vi "含算法图_new3.vi"() -> ()   [LabVIEW 2014]
uses:
  <vilib>/Instr/_visa.llb/VISA Configure Serial Port (Instr).vi
  test_last/Debug/test_last.dll
panel:
  out "数值 5":u8
  out "数值":dbl
  in  "?":enum32{"串口助手", "姿态界面", "曲线显示", "图像显示", "使用说明"}(tab)=enum."图像显示"
  in  "单选按钮":T1(radio)
  in  "?":bool
  out "接受数据个数":u32
  out "发送数据个数":u32
  in  "?":bool
  out "?":bool
  in  "?":bool
  in  "停止位":u16(ring)=10 items=["1.0"=10, "1.5"=15, "2.0"=20]
  in  "com口":refnum<visa-resource-name>="COM2"
  in  "波特率":u32(ring)=115200 items=["4800"=4800, "9600"=9600, "14400"=14400, "19200"=19200, "38400"=38400, "56000"=56000, "57600"=57600, "115200"=115200]
  in  "数据位数":u16(ring)=8 caption="数据位" items=["5"=5, "6"=6, "7"=7, "8"=8]
  in  "校验位":u16(ring) items=["None", "Odd", "Even", "Mark", "Space"]
  in  "?":string
  out "?":string
  in  "?":bool=TRUE
  out "数值 3":dbl
  out "数值 2":u8
  in  "舵机":sgl(slide) scale=5.0..10.0
  in  "电机":sgl(slide) scale=0.0..100.0
  out "数值 4":dbl
  out "波形图表":cluster{sgl, sgl}[](graph)
  in  "白界":u8=120
  in  "黑界":u8=100
  in  "列数":i32=190
  in  "行数":i32=130
  out "?":string
  out "new picture":picture caption="新图片"
  out "一帧数据数":i32
  in  "?":bool=TRUE
  # "数据类型"
  # "串口配置"
  # "串口号"
  # "上位机通信协议及功能介绍"
  # "功能1：串口助手"
  # "HEX:字符串显示\nDefault:十进制显示\nuint8:十六进制显示\nint32:输入字符串“in32”+BYTE1+BYTE2+BYTE3+BYTE4\nfloat:输入字符串“flot”+BYTE1+BYTE2+BYTE3+BYTE4\nuint32:输入字符串“ui32”+BYTE1+BYTE2+BYTE3+BYTE4"
  # "功能2：姿态界面"
  # "舵机发送：0x08+0x00+0x02+0x03+BYTE1+BYTE2+BYTE3+BYTE4\n电机发送：0X08+0X01+0X02+0X03+BYTE1+BYTE2+BYTE3+BYTE4"
  # "功能3：曲线显示"
  # "曲线1：“lin1”+BYTE1+BYTE2+BYTE3+BYTE4(发送一个float数据)\n曲线2：“lin2”+BYTE1+BYTE2+BYTE3+BYTE4(发送一个float数据)"
  # "功能4：图像显示"
  # "图像：发送字符串“image”+图像数组"
  # "LJ     HNU"
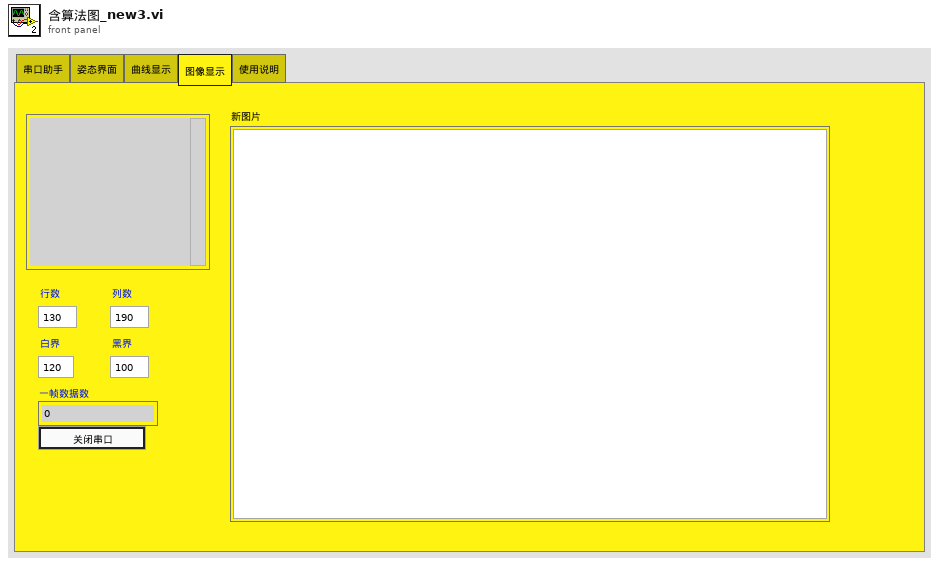
[diagram p1: front panel]
types:
  T1 = enum32{"uint8", "uint32", "HEX", "int8", "int32", "float", "Default"}
  T2 = typedef "imagedata.ctl" = cluster{"image type":i32, "image depth":i32, "image":u8[], "mask":u8[], "colors":u32[], "Rectangle":cluster{"left":i16, "top":i16, "right":i16, "bottom":i16}}
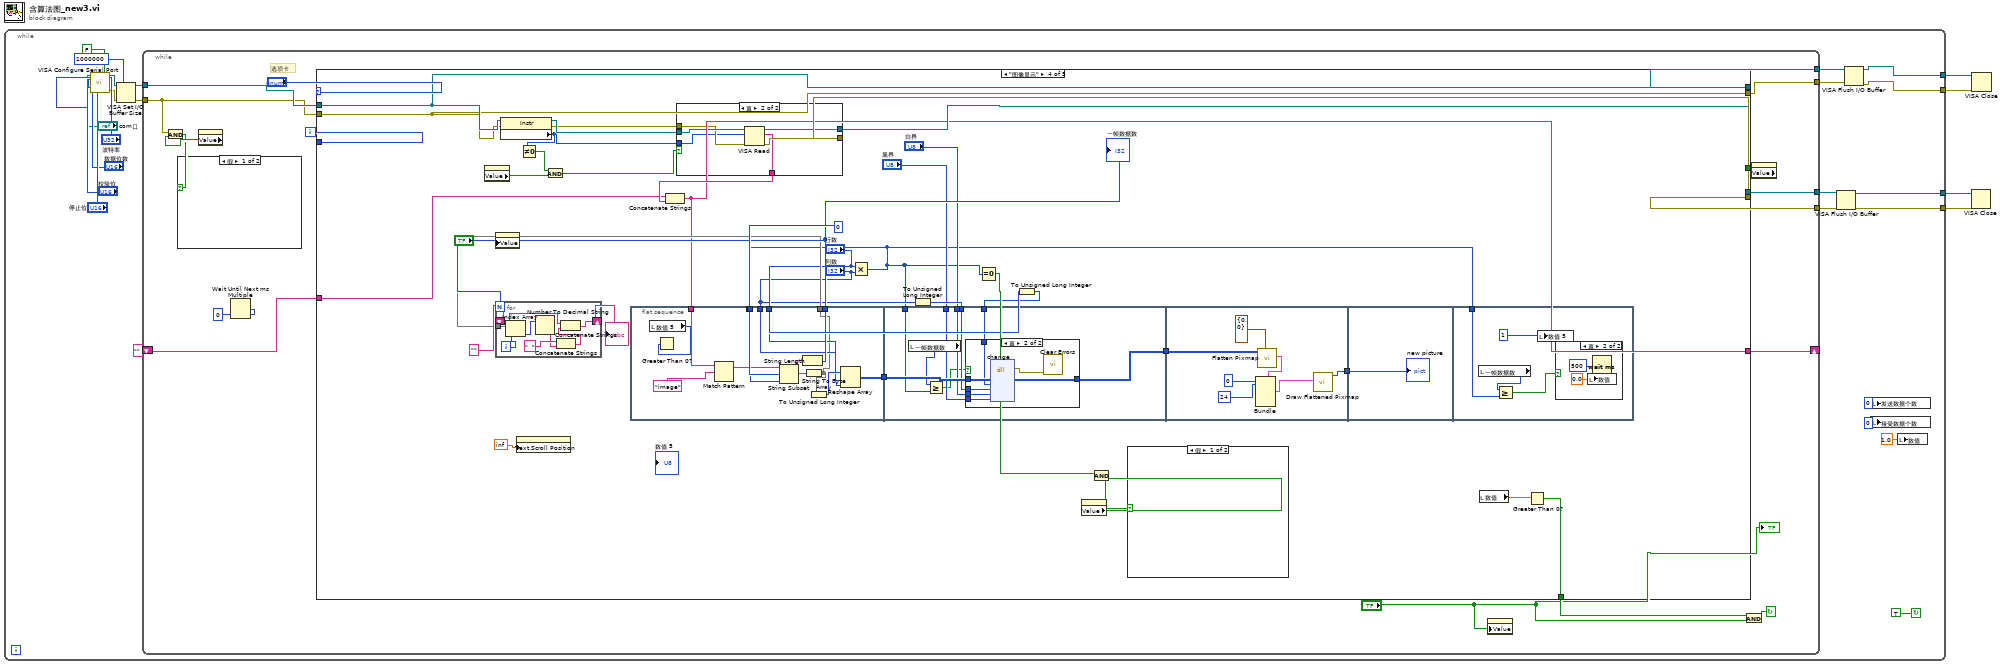
[diagram p0: block diagram]
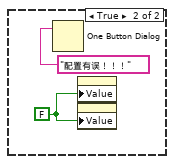
[diagram p2: hidden frame]
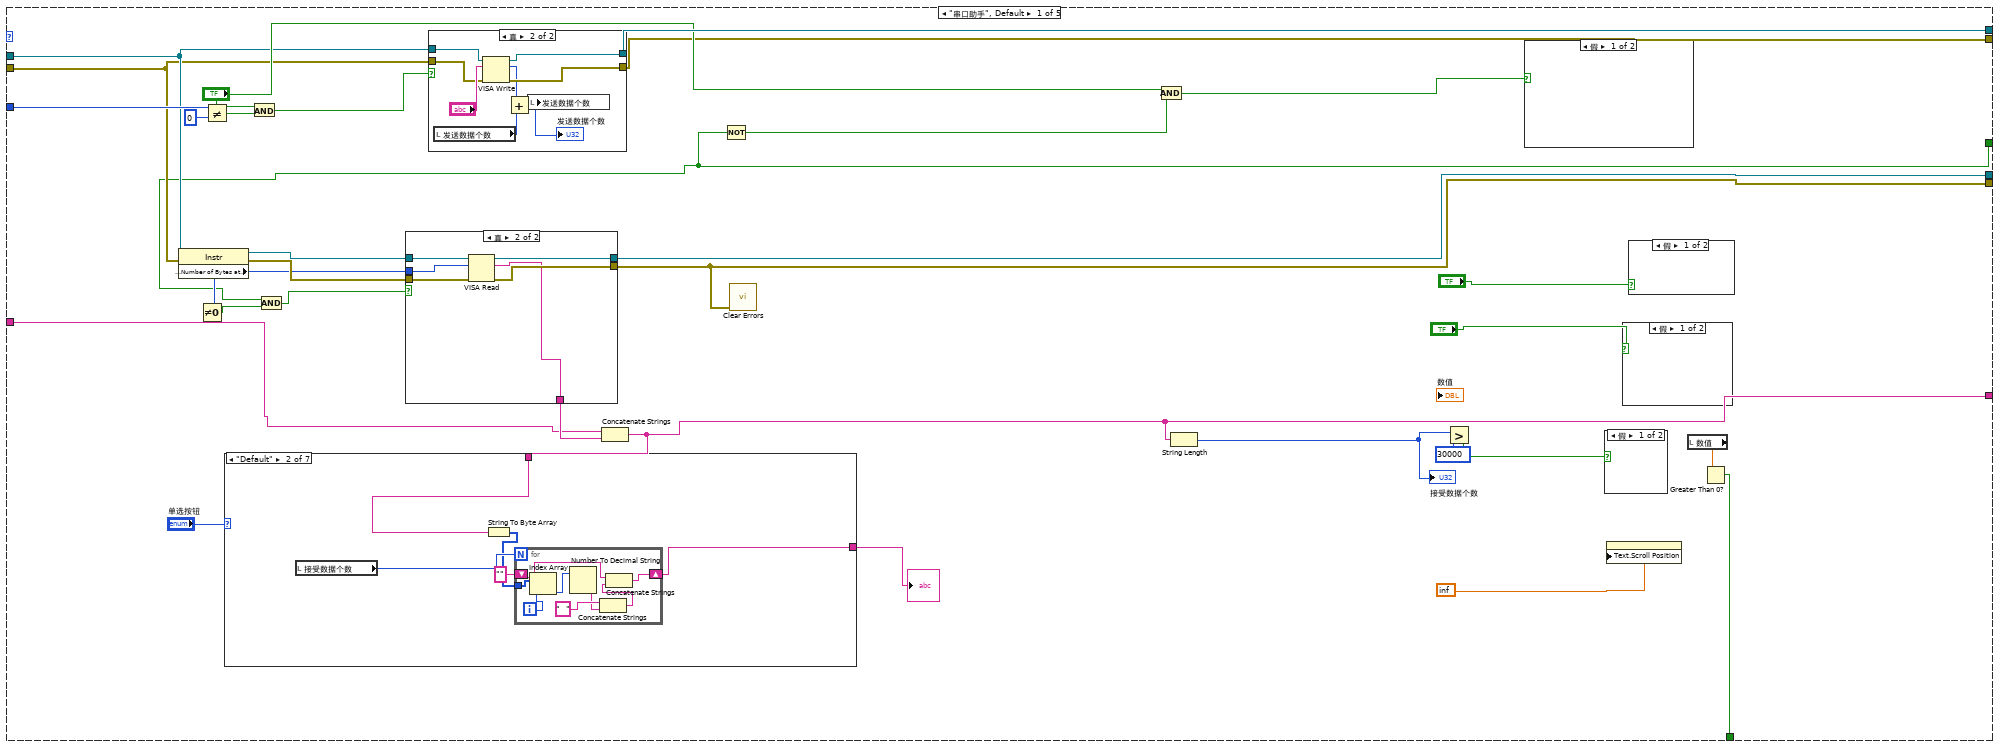
[diagram p3: hidden frame]
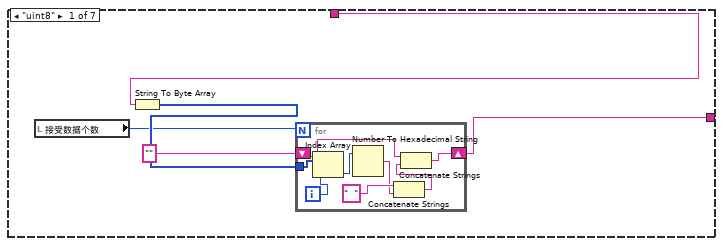
[diagram p4: hidden frame]
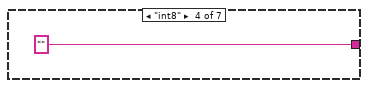
[diagram p6: hidden frame]
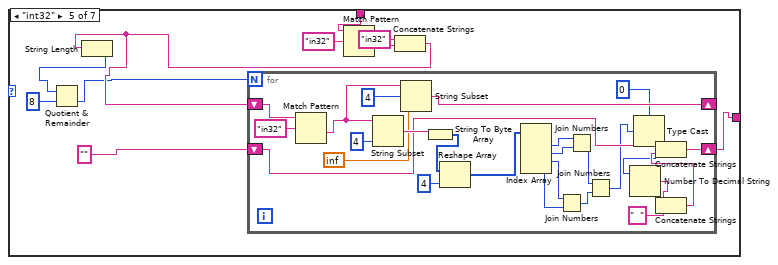
[diagram p7: hidden frame]
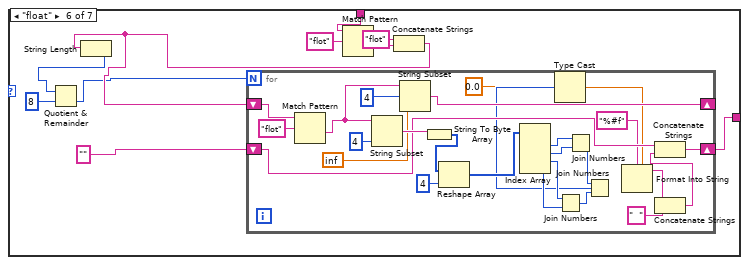
[diagram p8: hidden frame]
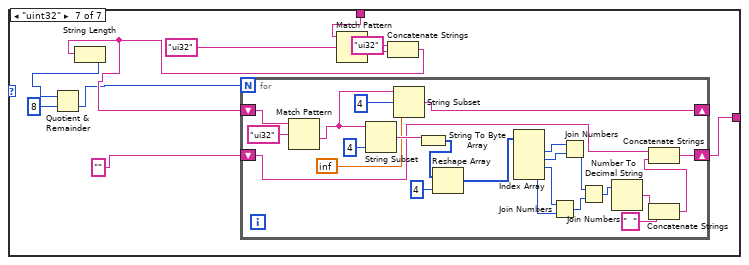
[diagram p9: hidden frame]
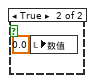
[diagram p10: hidden frame]
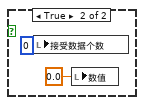
[diagram p11: hidden frame]
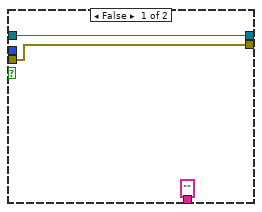
[diagram p12: hidden frame]
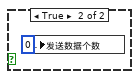
[diagram p13: hidden frame]
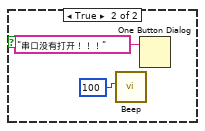
[diagram p14: hidden frame]
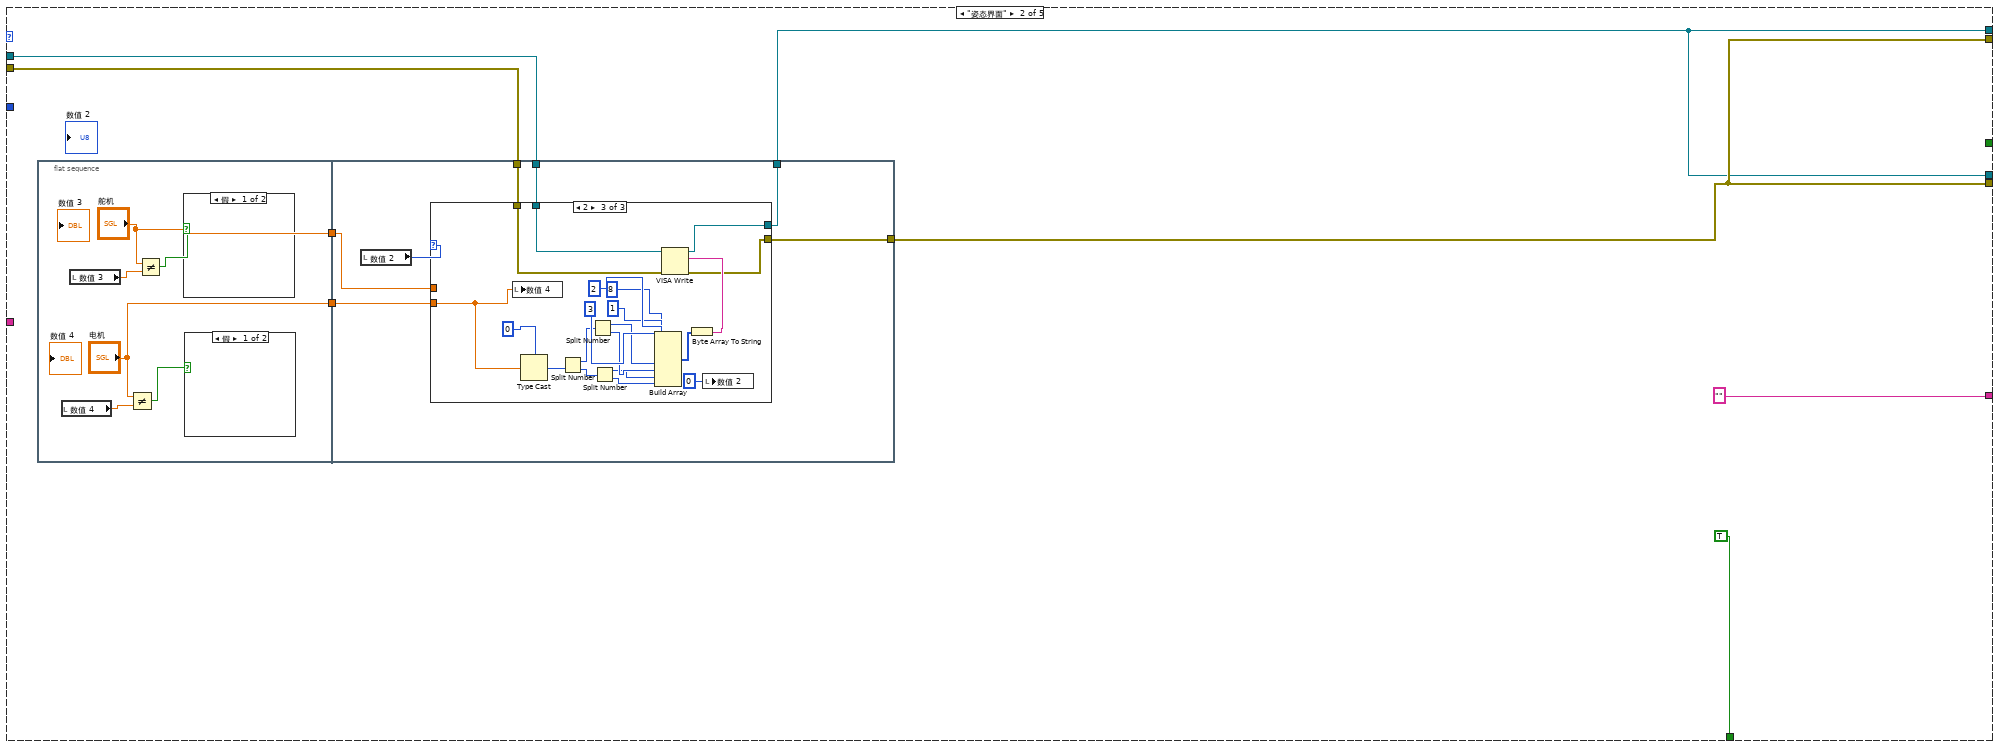
[diagram p16: hidden frame]
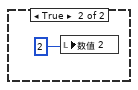
[diagram p17: hidden frame]
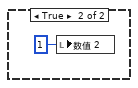
[diagram p18: hidden frame]
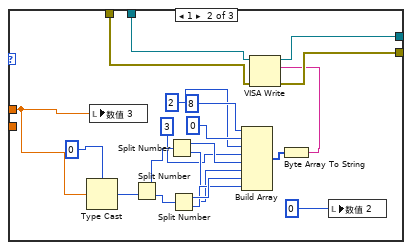
[diagram p20: hidden frame]
diagram:
  n1 = while {
    tunnel: [w9] -> w4
    tunnel: [w8] -> w3
    tunnel: [w7] -> w2
    tunnel: [w6] -> w1
    stop <- TRUE continue-if-true
    n2 = call-poly "VISA Configure Serial Port"("VISA resource name"="com口", "Enable Termination\nChar (T)"=FALSE ("Enable Termination\nChar (T)"), "baud rate (9600)"="波特率", "data bits (8)"="数据位数", "parity (0:none)"="校验位", "stop bits (10: 1 bit)"="停止位") -> ("VISA resource name out"=w22:refnum<visa-resource-name>, "error out"=w20:errorcluster)  [unwired: 8 in]
    n3 = VISA Set I/O Buffer Size(VISA resource name=w22, size (4096)=1000000, error in (no error)=w20) -> (VISA resource name out=w15:refnum<visa-resource-name>, error out=w5:errorcluster)  [unwired: 1 in]
    n4 = while {
      tunnel: w15 -> [w43]
      tunnel: w5 -> [w32]
      shift-right: [w42] -> _
      shift-left: "" -> [w41]
      tunnel: [w36] -> w14
      tunnel: [w33] -> w13
      tunnel: [w35] -> w12
      tunnel: [w34] -> w11
      i -> [w45]
      stop <- w39 continue-if-true
      # "选项卡"
      n5 = property class="Bool (严格)"() -> ("Value"=w31:bool)  [unwired: 2 in, 2 out]
      n6 = And(x=w32, y=w31) -> (x .and. y?=w30:bool)
      n7 = case shown="假" w30 {
        frame False {
        }
        frame True {
          w46 = FALSE
          n8 = One Button Dialog(message="配置有误！！！" ("消息")) -> ()  [unwired: 1 in, 1 out]
          n9 = property class="Bool (严格)"("Value"=w46) -> ()  [unwired: 2 in, 2 out]
          n10 = property class="Bool (严格)"("Value"=w46) -> ()  [unwired: 2 in, 2 out]
        }
      }
      n11 = Wait Until Next ms Multiple(millisecond multiple=u32 0 ("毫秒倍数")) -> ()  [unwired: 1 out]
      n12 = property class="Bool (严格)"("Value"="?") -> ()  [unwired: 2 in, 2 out]
      n13 = property class="Bool (严格)"() -> ("Value"=w37:bool)  [unwired: 2 in, 2 out]
      n14 = case shown="\"图像显示\"" "?" {
        tunnel: [w79 w237 w324 w416 w484] -> w36
        tunnel: [w49 w238 w323 w395 w483] -> w33
        tunnel: w45 -> [w78 _ _ _ _]
        tunnel: w43 -> [w70 w241 w331 w416 w484]
        tunnel: w32 -> [w69 w240 w330 w395 w483]
        tunnel: w37 -> [w59 _ _ _ _]
        tunnel: [w65 w237 w324 w415 w484] -> w35
        tunnel: [w48 w238 w323 w417 w483] -> w34
        tunnel: [w50 "" "" w384 ""] -> w42
        tunnel: w41 -> [w60 _ w319 w405 _]
        tunnel: [w62 TRUE TRUE w407 TRUE] -> w40
        frame "串口助手", Default {
          n15 = property class="Instr"(reference=w70, error in=w69) -> (reference out=w68:refnum<visa-resource-name>, error out=w67:errorcluster, "Serial Settings:Number of Bytes at Serial Port"=w66:u32)
          n16 = Not Equal To 0?(x=w66) -> (x != 0?=w58:bool)
          n17 = Not Equal?(x=w78, y=0) -> (x != y?=w76:bool)
          n18 = And(x="?", y=w76) -> (x .and. y?=w75:bool)
          n19 = And(x=w59, y=w58) -> (x .and. y?=w57:bool)
          n20 = case shown="真" w57 {
            tunnel: w68 -> [w217 w223]
            tunnel: w67 -> [w216 w222]
            tunnel: w66 -> [_ w221]
            tunnel: [w217 w220] -> w65
            tunnel: [w216 w219] -> w48
            tunnel: ["" ("read buffer") w218] -> w61
            frame False {
            }
            frame True {
              n21 = VISA Read(VISA resource name=w223, byte count=w221, error in (no error)=w222) -> (VISA resource name out=w220:refnum<visa-resource-name>, read buffer=w218:string, error out=w219:errorcluster)  [unwired: 1 out]
            }
          }
          n22 = case shown="真" w75 {
            tunnel: [w228 w236] -> w79
            tunnel: [w227 w234] -> w49
            tunnel: w70 -> [w228 w233]
            tunnel: w69 -> [w227 w232]
            frame False {
            }
            frame True {
              n23 = local read "发送数据个数"() -> (w230:u32)
              n24 = VISA Write(VISA resource name=w233, write buffer="?", error in (no error)=w232) -> (VISA resource name out=w236:refnum<visa-resource-name>, return count=w231:u32, error out=w234:errorcluster)
              n25 = Add(x=w231, y=w230) -> (x+y=w229:u32)
              "发送数据个数" <- w229
              n26 = local write "发送数据个数"(w229) -> ()
            }
          }
          n27 = Concatenate Strings(w60, w61) -> (w50:string)
          n28 = case shown="\"Default\"" "单选按钮" {
            tunnel: [w80 w95 w106 "" w108 w147 w188] -> w51
            tunnel: w50 -> [w81 w93 w106 _ w109 w146 w186]
            frame "uint8" {
              n29 = local read "接受数据个数"() -> (w82:u32)
              n30 = String To Byte Array(string=w81) -> (unsigned byte array=w84:u8[])
              n31 = for {
                N: w82 -> [_]
                tunnel: w84 -> [w91]
                shift-right: [w90] -> w80
                shift-left: "" -> [w89]
                i -> [w92]
                n32 = Index Array(array=w91, index=w92) -> (element=w86:u8)
                n33 = Number To Hexadecimal String(2:w86) -> (0:w85:string)  [unwired: 1 in]
                n34 = Concatenate Strings("  " ("字符串"), w85) -> (w88:string)
                n35 = Concatenate Strings(w89, w88) -> (w90:string)
              }
            }
            frame "Default" {
              n36 = local read "接受数据个数"() -> (w97:u32)
              n37 = String To Byte Array(string=w93) -> (unsigned byte array=w96:u8[])
              n38 = for {
                N: w97 -> [_]
                tunnel: w96 -> [w104]
                shift-right: [w102] -> w95
                shift-left: "" -> [w101]
                i -> [w105]
                n39 = Index Array(array=w104, index=w105) -> (element=w103:u8)
                n40 = Number To Decimal String(number=w103) -> (decimal integer string=w98:string)  [unwired: 1 in]
                n41 = Concatenate Strings("  " ("字符串"), w98) -> (w100:string)
                n42 = Concatenate Strings(w101, w100) -> (w102:string)
              }
            }
            frame "HEX", Default {
            }
            frame "int8" {
            }
            frame "int32" {
              n43 = Match Pattern(string=w109, regular expression="in32" ("正则表达式")) -> (after substring=w115:string)  [unwired: 1 in, 3 out]
              n44 = Concatenate Strings("in32" ("字符串"), w115) -> (w113:string)
              n45 = String Length(string=w113) -> (length=w112:i32)
              n46 = Quotient & Remainder(x=w112, y=8) -> (floor(x/y)=w110:i32)  [unwired: 1 out]
              n47 = for {
                N: w110 -> [_]
                shift-right: [w125] -> _
                shift-left: w113 -> [w138]
                shift-right: [w124] -> w108
                shift-left: "" -> [w123]
                n48 = Match Pattern(string=w138, regular expression="in32" ("正则表达式")) -> (after substring=w128:string)  [unwired: 1 in, 3 out]
                n49 = String Subset(string=w128, length (rest)=4 ("长度（剩余）")) -> (substring=w135:string)  [unwired: 1 in]
                n50 = String Subset(string=w128, offset (0)=4, length (rest)=inf) -> (substring=w125:string)
                n51 = String To Byte Array(string=w135) -> (unsigned byte array=w134:u8[])
                n52 = Reshape Array(w134, 4 ("维数大小")) -> (w122:u8[])
                n53 = Index Array(array=w122) -> (element #1=w132:u8, element #2=w131:u8, element #3=w130:u8, element #4=w129:u8)  [unwired: 4 in]
                n54 = Join Numbers(hi=w130, lo=w129) -> ((hi.lo)=w141:u16)
                n55 = Join Numbers(hi=w132, lo=w131) -> ((hi.lo)=w142:u16)
                n56 = Join Numbers(hi=w142, lo=w141) -> ((hi.lo)=w121:u32)
                n57 = Type Cast(type=0, x=w121) -> (*(type *) &x=w119:i32)
                n58 = Number To Decimal String(number=w119) -> (decimal integer string=w118:string)  [unwired: 1 in]
                n59 = Concatenate Strings(w118, "  " ("字符串")) -> (w139:string)
                n60 = Concatenate Strings(w123, w139) -> (w124:string)
              }
            }
            frame "float" {
              n61 = Match Pattern(string=w146, regular expression="flot" ("正则表达式")) -> (after substring=w150:string)  [unwired: 1 in, 3 out]
              n62 = Concatenate Strings("flot" ("字符串"), w150) -> (w148:string)
              n63 = String Length(string=w148) -> (length=w145:i32)
              n64 = Quotient & Remainder(x=w145, y=8) -> (floor(x/y)=w143:i32)  [unwired: 1 out]
              n65 = for {
                N: w143 -> [_]
                shift-right: [w161] -> _
                shift-left: w148 -> [w174]
                shift-right: [w160] -> w147
                shift-left: "" -> [w159]
                n66 = Match Pattern(string=w174, regular expression="flot" ("正则表达式")) -> (after substring=w164:string)  [unwired: 1 in, 3 out]
                n67 = String Subset(string=w164, length (rest)=4 ("长度（剩余）")) -> (substring=w171:string)  [unwired: 1 in]
                n68 = String Subset(string=w164, offset (0)=4, length (rest)=inf) -> (substring=w161:string)
                n69 = String To Byte Array(string=w171) -> (unsigned byte array=w170:u8[])
                n70 = Reshape Array(w170, 4 ("维数大小")) -> (w158:u8[])
                n71 = Index Array(array=w158) -> (element #1=w168:u8, element #2=w167:u8, element #3=w166:u8, element #4=w165:u8)  [unwired: 4 in]
                n72 = Join Numbers(hi=w166, lo=w165) -> ((hi.lo)=w177:u16)
                n73 = Join Numbers(hi=w168, lo=w167) -> ((hi.lo)=w178:u16)
                n74 = Join Numbers(hi=w178, lo=w177) -> ((hi.lo)=w157:u32)
                n75 = Type Cast(type=sgl 0.0, x=w157) -> (*(type *) &x=w155:sgl)
                n76 = Format Into String(format string="%#f" ("初始字符串"), w155) -> (resulting string=w154:string)  [unwired: 2 in, 1 out]
                n77 = Concatenate Strings(w154, "  " ("字符串")) -> (w175:string)
                n78 = Concatenate Strings(w159, w175) -> (w160:string)
              }
            }
            frame "uint32" {
              n79 = Match Pattern(string=w186, regular expression="ui32" ("正则表达式")) -> (after substring=w184:string)  [unwired: 1 in, 3 out]
              n80 = Concatenate Strings("ui32" ("字符串"), w184) -> (w182:string)
              n81 = String Length(string=w182) -> (length=w181:i32)
              n82 = Quotient & Remainder(x=w181, y=8) -> (floor(x/y)=w179:i32)  [unwired: 1 out]
              n83 = for {
                N: w179 -> [_]
                shift-right: [w191] -> _
                shift-left: w182 -> [w205]
                shift-right: [w190] -> w188
                shift-left: "" -> [w189]
                n84 = Match Pattern(string=w205, regular expression="ui32" ("正则表达式")) -> (after substring=w194:string)  [unwired: 1 in, 3 out]
                n85 = String Subset(string=w194, length (rest)=4 ("长度（剩余）")) -> (substring=w202:string)  [unwired: 1 in]
                n86 = String Subset(string=w194, offset (0)=4, length (rest)=inf) -> (substring=w191:string)
                n87 = String To Byte Array(string=w202) -> (unsigned byte array=w201:u8[])
                n88 = Reshape Array(w201, 4 ("维数大小")) -> (w199:u8[])
                n89 = Index Array(array=w199) -> (element #1=w198:u8, element #2=w197:u8, element #3=w196:u8, element #4=w195:u8)  [unwired: 4 in]
                n90 = Join Numbers(hi=w196, lo=w195) -> ((hi.lo)=w210:u16)
                n91 = Join Numbers(hi=w198, lo=w197) -> ((hi.lo)=w211:u16)
                n92 = Join Numbers(hi=w211, lo=w210) -> ((hi.lo)=w209:u32)
                n93 = Number To Decimal String(number=w209) -> (decimal integer string=w208:string)  [unwired: 1 in]
                n94 = Concatenate Strings(w208, "  " ("字符串")) -> (w206:string)
                n95 = Concatenate Strings(w189, w206) -> (w190:string)
              }
            }
          }
          "?" <- w51
          n96 = Not(x=w59) -> (.not. x?=w74:bool)
          n97 = call <vilib>:"Clear Errors.vi"("error in (no error)"=w48) -> ()  [unwired: 5 in, 2 out]
          n98 = And(x="?", y=w74) -> (x .and. y?=w72:bool)
          n99 = String Length(string=w50) -> (length=w56:i32)
          "接受数据个数" <- w56
          n100 = Greater?(x=w56, y=u32 30000) -> (0:w54:bool)
          n101 = case shown="假" w72 {
            frame False {
            }
            frame True {
              n102 = call <vilib>:"Beep.vi"("duration (msec)"=100) -> ()  [unwired: 11 in]
              n103 = One Button Dialog(message="串口没有打开！！！" ("消息")) -> ()  [unwired: 1 in, 1 out]
            }
          }
          n104 = case shown="假" w54 {
            frame False {
            }
            frame True {
              n105 = local write "数值"(0.0 ("数值")) -> ()
            }
          }
          n106 = property class="Str"("Text.Scroll Position"=inf) -> ()  [unwired: 2 in, 2 out]
          n107 = case shown="假" "?" {
            frame False {
            }
            frame True {
              n108 = local write "接受数据个数"(u32 0 ("接受数据个数")) -> ()
              n109 = local write "数值"(0.0 ("数值")) -> ()
            }
          }
          n110 = case shown="假" "?" {
            frame False {
            }
            frame True {
              n111 = local write "发送数据个数"(u32 0 ("数据个数")) -> ()
            }
          }
          n112 = local read "数值"() -> (w63:dbl)
          n113 = Greater Than 0?(x=w63) -> (x > 0?=w62:bool)
        }
        frame "姿态界面" {
          n114 = flat-sequence {
            tunnel: ["舵机"] -> w242
            tunnel: ["电机"] -> w239
            tunnel: w242 -> [w258]
            tunnel: w241 -> [w257]
            tunnel: w240 -> [w256]
            tunnel: w239 -> [w255]
            tunnel: [w254] -> w237
            tunnel: [w253] -> w238
            frame #0 {
              n115 = local read "数值 4"() -> (w246:dbl)
              n116 = local read "数值 3"() -> (w247:dbl)
              n117 = Not Equal?(x="电机", y=w246) -> (x != y?=w248:bool)
              n118 = Not Equal?(x="舵机", y=w247) -> (x != y?=w249:bool)
              n119 = case shown="假" w249 {
                frame False {
                }
                frame True {
                  n120 = local write "数值 2"(u8 1 ("数值 2")) -> ()
                }
              }
              n121 = case shown="假" w248 {
                frame False {
                }
                frame True {
                  n122 = local write "数值 2"(u8 2 ("数值 2")) -> ()
                }
              }
            }
            frame #1 {
              n123 = local read "数值 2"() -> (w259:u8)
              n124 = case shown="2" w259 {
                tunnel: [w261 w281 w287] -> w254
                tunnel: [w260 w280 w286] -> w253
                tunnel: w258 -> [_ w265 _]
                tunnel: w257 -> [w261 w264 w285]
                tunnel: w256 -> [w260 w263 w284]
                tunnel: w255 -> [_ _ w283]
                frame 0, Default {
                }
                frame 1 {
                  n125 = Type Cast(type=0, x=w265) -> (*(type *) &x=w266:i32)
                  n126 = local write "数值 3"(w265) -> ()
                  n127 = Split Number(x=w266) -> (hi(x)=w279:u16, lo(x)=w278:u16)
                  n128 = Split Number(x=w279) -> (hi(x)=w273:u8, lo(x)=w274:u8)
                  n129 = Split Number(x=w278) -> (hi(x)=w276:u8, lo(x)=w275:u8)
                  n130 = Build Array(8, 0, 2, 3, w273, w274, w276, w275) -> (w268:i32[])
                  n131 = Byte Array To String(unsigned byte array=w268) -> (string=w277:string)
                  n132 = VISA Write(VISA resource name=w264, write buffer=w277, error in (no error)=w263) -> (VISA resource name out=w281:refnum<visa-resource-name>, error out=w280:errorcluster)  [unwired: 1 out]
                  n133 = local write "数值 2"(u8 0 ("数值 2")) -> ()
                }
                frame 2 {
                  n134 = local write "数值 4"(w283) -> ()
                  n135 = Type Cast(type=0, x=w283) -> (*(type *) &x=w301:i32)
                  n136 = Split Number(x=w301) -> (hi(x)=w288:u16, lo(x)=w289:u16)
                  n137 = Split Number(x=w288) -> (hi(x)=w294:u8, lo(x)=w293:u8)
                  n138 = Split Number(x=w289) -> (hi(x)=w291:u8, lo(x)=w292:u8)
                  n139 = Build Array(8, 1, 2, 3, w294, w293, w291, w292) -> (w299:i32[])
                  n140 = Byte Array To String(unsigned byte array=w299) -> (string=w290:string)
                  n141 = VISA Write(VISA resource name=w285, write buffer=w290, error in (no error)=w284) -> (VISA resource name out=w287:refnum<visa-resource-name>, error out=w286:errorcluster)  [unwired: 1 out]
                  n142 = local write "数值 2"(u8 0 ("数值 2")) -> ()
                }
              }
            }
          }
        }
        frame "曲线显示" {
          n143 = property class="Bool (严格)"() -> ("Value"=w329:bool)  [unwired: 2 in, 2 out]
          n144 = property class="Instr"(reference=w331, error in=w330) -> (reference out=w326:refnum<visa-resource-name>, error out=w325:errorcluster, "Serial Settings:Number of Bytes at Serial Port"=w327:u32)
          n145 = Not Equal To 0?(x=w327) -> (x != 0?=w332:bool)
          n146 = And(x=w329, y=w332) -> (x .and. y?=w328:bool)
          n147 = case shown="真" w328 {
            tunnel: w327 -> [_ w382]
            tunnel: w326 -> [w376 w381]
            tunnel: w325 -> [w375 w380]
            tunnel: [w376 w379] -> w324
            tunnel: [w375 w378] -> w323
            tunnel: ["" ("read buffer") w377] -> w317
            frame False {
            }
            frame True {
              n148 = VISA Read(VISA resource name=w381, byte count=w382, error in (no error)=w380) -> (VISA resource name out=w379:refnum<visa-resource-name>, read buffer=w377:string, error out=w378:errorcluster)  [unwired: 1 out]
            }
          }
          n149 = Concatenate Strings(w319, w317) -> (w318:string)
          n150 = Match Pattern(string=w318, regular expression="lin" ("正则表达式")) -> (after substring=w321:string)  [unwired: 1 in, 3 out]
          n151 = Concatenate Strings("lin" ("字符串"), w321) -> (w306:string)
          n152 = Search and Replace String(replace all?=TRUE ("替换全部？(F)"), input string=w306, search string="lin2" ("替换字符串(\"\")"), replace string="lin2" ("搜索字符串")) -> (number of replacements=w308:i32)  [unwired: 4 in, 3 out]
          n153 = Search and Replace String(replace all?=TRUE ("替换全部？(F)"), input string=w306, search string="lin1" ("替换字符串(\"\")"), replace string="lin1" ("搜索字符串")) -> (number of replacements=w313:i32)  [unwired: 4 in, 3 out]
          n154 = Decrement(x=w308) -> (x-1=w311:i32)
          n155 = Decrement(x=w313) -> (x-1=w316:i32)
          n156 = for {
            N: w316 -> [_]
            shift-right: [w358] -> _
            shift-left: w306 -> [w371]
            tunnel: [w354] -> w305 mode=indexing
            n157 = Match Pattern(string=w371, regular expression="lin1" ("正则表达式")) -> (after substring=w361:string)  [unwired: 1 in, 3 out]
            n158 = String Subset(string=w361, length (rest)=4 ("长度（剩余）")) -> (substring=w368:string)  [unwired: 1 in]
            n159 = String Subset(string=w361, offset (0)=4, length (rest)=inf) -> (substring=w358:string)
            n160 = String To Byte Array(string=w368) -> (unsigned byte array=w367:u8[])
            n161 = Reshape Array(w367, 4 ("维数大小")) -> (w357:u8[])
            n162 = Index Array(array=w357) -> (element #1=w365:u8, element #2=w364:u8, element #3=w363:u8, element #4=w362:u8)  [unwired: 4 in]
            n163 = Join Numbers(hi=w363, lo=w362) -> ((hi.lo)=w372:u16)
            n164 = Join Numbers(hi=w365, lo=w364) -> ((hi.lo)=w373:u16)
            n165 = Join Numbers(hi=w373, lo=w372) -> ((hi.lo)=w356:u32)
            n166 = Type Cast(type=sgl 0.0, x=w356) -> (*(type *) &x=w354:sgl)
          }
          n167 = for {
            N: w311 -> [_]
            shift-right: [w338] -> _
            shift-left: w306 -> [w351]
            tunnel: [w334] -> w304 mode=indexing
            n168 = Match Pattern(string=w351, regular expression="lin2" ("正则表达式")) -> (after substring=w341:string)  [unwired: 1 in, 3 out]
            n169 = String Subset(string=w341, length (rest)=4 ("长度（剩余）")) -> (substring=w348:string)  [unwired: 1 in]
            n170 = String Subset(string=w341, offset (0)=4, length (rest)=inf) -> (substring=w338:string)
            n171 = String To Byte Array(string=w348) -> (unsigned byte array=w347:u8[])
            n172 = Reshape Array(w347, 4 ("维数大小")) -> (w337:u8[])
            n173 = Index Array(array=w337) -> (element #1=w345:u8, element #2=w344:u8, element #3=w343:u8, element #4=w342:u8)  [unwired: 4 in]
            n174 = Join Numbers(hi=w343, lo=w342) -> ((hi.lo)=w352:u16)
            n175 = Join Numbers(hi=w345, lo=w344) -> ((hi.lo)=w353:u16)
            n176 = Join Numbers(hi=w353, lo=w352) -> ((hi.lo)=w336:u32)
            n177 = Type Cast(type=sgl 0.0, x=w336) -> (*(type *) &x=w334:sgl)
          }
          n178 = Build Cluster Array(w305, w304) -> (→"波形图表":cluster{sgl, sgl}[])
        }
        frame "图像显示" {
          n179 = property class="Bool (严格)"() -> ("Value"=w409:bool)  [unwired: 2 in, 2 out]
          n180 = property class="Bool (严格)"("Value"="?") -> ()  [unwired: 2 in, 2 out]
          n181 = for {
            N: w400 -> [_]
            shift-right: [w470] -> w403
            shift-left: "" -> [w469]
            tunnel: w394 -> [w465]
            i -> [w471]
            n182 = Index Array(array=w465, index=w471) -> (element=w464:u8)
            n183 = Number To Decimal String(number=w464) -> (decimal integer string=w466:string)  [unwired: 1 in]
            n184 = Concatenate Strings("  " ("字符串"), w466) -> (w468:string)
            n185 = Concatenate Strings(w469, w468) -> (w470:string)
          }
          "?" <- w403
          n186 = property class="Instr"(reference=w416, error in=w395) -> (reference out=w414:refnum<visa-resource-name>, error out=w413:errorcluster, "Serial Settings:Number of Bytes at Serial Port"=w412:u32)
          n187 = property class="Str"("Text.Scroll Position"=inf) -> ()  [unwired: 2 in, 2 out]
          n188 = Not Equal To 0?(x=w412) -> (x != 0?=w411:bool)
          n189 = And(x=w411, y=w409) -> (x .and. y?=w410:bool)
          n190 = flat-sequence {
            tunnel: 0 ("偏移量(0)") -> [w430]
            tunnel: [w427] -> w400
            tunnel: w383 -> [w426]
            tunnel: [w419] -> w394
            tunnel: "行数" -> [w424]
            tunnel: "列数" -> [w423]
            tunnel: [w422] -> w391
            tunnel: w384 -> [w420]
            tunnel: w391 -> [w439]
            tunnel: w390 -> [w438]
            tunnel: w389 -> [w437]
            tunnel: "白界" -> [w436]
            tunnel: "黑界" -> [w435]
            tunnel: [w434] -> w386
            tunnel: w383 -> [w432]
            tunnel: w386 -> [w453]
            tunnel: [w448] -> w385
            tunnel: w385 -> [w455]
            tunnel: w383 -> [w457]
            frame #0 {
              n191 = local read "数值 5"() -> (w418:u8)
              n192 = Greater Than 0?(x=w418) -> ()  [unwired: 1 out]
              n193 = Match Pattern(string=w420, regular expression="image" ("正则表达式")) -> (after substring=w429:string)  [unwired: 1 in, 3 out]
              n194 = String Subset(string=w429, offset (0)=w430, length (rest)=w426) -> (substring=w428:string)
              n195 = String Length(string=w428) -> (length=w427:i32)
              n196 = String To Byte Array(string=w428) -> (unsigned byte array=w419:u8[])
              n197 = To Unsigned Long Integer(number=w419) -> (unsigned 32bit integer=w425:u32[])
              n198 = Reshape Array(w425, w424, w423) -> (w422:u32[][])
            }
            frame #1 {
              n199 = local read "一帧数据数"() -> (w433:i32)
              n200 = Greater Or Equal?(x=w433, y=w432) -> (x >= y?=w431:bool)
              n201 = case shown="真" w431 {
                tunnel: w439 -> [_ w447]
                tunnel: w438 -> [_ w446]
                tunnel: w437 -> [_ w445]
                tunnel: w436 -> [_ w444]
                tunnel: w435 -> [_ w443]
                tunnel: [u32[][] [] ("date") w442] -> w434
                frame False {
                }
                frame True {
                  n202 = dll-call lib="C:/Users/love  ben/Desktop/NI/test_last/Debug/test_last.dll" fn="change"("date"=w447, "hang"=w445, "lie"=w446, "white"=w444, "dark"=w443) -> (error out=w441:errorcluster, "date"=w442:u32[][])  [unwired: 8 in, 1 out]
                  n203 = call <vilib>:"Clear Errors.vi"("error in (no error)"=w441) -> ()  [unwired: 5 in, 2 out]
                }
              }
            }
            frame #2 {
              n204 = call <vilib>:"Flatten Pixmap.vi"("top left"=cluster{"x":i16, "y":i16} {"x"=0, "y"=0}, "24-bit pixmap"=w453) -> ("image data"=w452:T2)  [unwired: 9 in]
              n205 = Bundle(cluster=w452, "image type"=0, "image depth"=24) -> (w449:T2)  [unwired: 4 in]
              n206 = call <vilib>:"Draw Flattened Pixmap.vi"("image data"=w449) -> ("new picture"=w448:picture)  [unwired: 8 in]
            }
            frame #3 {
              "new picture" <- w455
            }
            frame #4 {
              n207 = local read "一帧数据数"() -> (w459:i32)
              n208 = Greater Or Equal?(x=w459, y=w457) -> (x >= y?=w458:bool)
              n209 = local write "数值 5"(u8 1 ("数值 5")) -> ()
              n210 = case shown="真" w458 {
                frame False {
                }
                frame True {
                  n211 = local write "数值"(0.0 ("数值")) -> ()
                  n212 = Wait (ms)(milliseconds to wait=u32 500 ("等待时间（毫秒）")) -> ()  [unwired: 1 out]
                }
              }
            }
          }
          n213 = case shown="真" w410 {
            tunnel: w414 -> [w473 w480]
            tunnel: w413 -> [w474 w479]
            tunnel: [w474 w478] -> w417
            tunnel: [w473 w477] -> w415
            tunnel: w412 -> [_ w476]
            tunnel: ["" ("read buffer") w475] -> w406
            frame False {
            }
            frame True {
              n214 = VISA Read(VISA resource name=w480, byte count=w476, error in (no error)=w479) -> (VISA resource name out=w477:refnum<visa-resource-name>, read buffer=w475:string, error out=w478:errorcluster)  [unwired: 1 out]
            }
          }
          n215 = Concatenate Strings(w405, w406) -> (w384:string)
          n216 = Multiply(x="行数", y="列数") -> (x*y=w383:i32)
          n217 = To Unsigned Long Integer(number="列数") -> (unsigned 32bit integer=w390:u32)
          n218 = Equal To 0?(x=w383) -> (x = 0?=w398:bool)
          n219 = To Unsigned Long Integer(number="行数") -> (unsigned 32bit integer=w389:u32)
          n220 = property class="Bool (严格)"() -> ("Value"=w397:bool)  [unwired: 2 in, 2 out]
          n221 = And(x=w398, y=w397) -> (x .and. y?=w399:bool)
          n222 = case shown="假" w399 {
            frame False {
            }
            frame True {
              n223 = property class="Bool (严格)"("Value"=FALSE) -> ()  [unwired: 2 in, 2 out]
              n224 = One Button Dialog(message="请先设置正确参数！！！" ("消息")) -> ()  [unwired: 1 in, 1 out]
            }
          }
          n225 = local read "数值"() -> (w408:dbl)
          n226 = Greater Than 0?(x=w408) -> (x > 0?=w407:bool)
          "一帧数据数" <- w400
        }
        frame "使用说明" {
        }
      }
      n227 = And(x=w40, y="?") -> (x .and. y?=w39:bool)
      "?" <- "?"
    }
    n228 = VISA Flush I/O Buffer(VISA resource name=w12, error in (no error)=w11) -> (VISA resource name out=w7:refnum<visa-resource-name>, error out=w6:errorcluster)  [unwired: 1 in]
    n229 = VISA Flush I/O Buffer(VISA resource name=w14, error in (no error)=w13) -> (VISA resource name out=w9:refnum<visa-resource-name>, error out=w8:errorcluster)  [unwired: 1 in]
    n230 = local write "发送数据个数"(u32 0 ("数据个数")) -> ()
    n231 = local write "接受数据个数"(u32 0 ("接受数据个数")) -> ()
    n232 = local write "数值"(1.0 ("数值")) -> ()
  }
  n233 = VISA Close(VISA resource name=w2, error in (no error)=w1) -> ()  [unwired: 1 out]
  n234 = VISA Close(VISA resource name=w4, error in (no error)=w3) -> ()  [unwired: 1 out]
